vi "Open OPC UA Connection.vi"(8 "error in (no error)":errorcluster, 10 "OPC UA configuration":refnum<class "OPC UA configuration.lvclass">, 11 "OPC UA runtime in":refnum<class "OPC UA runtime.lvclass">) -> (0 "error out":errorcluster, 3 "OPC UA runtime out":refnum<class "OPC UA runtime.lvclass">)   [LabVIEW 2013, in "OPC UA runtime.lvclass"]
doc: "Opens connection to either an OPC UA Client or Server."
uses:
  OPC UA runtime.lvclass
  configuration/OPC UA configuration.lvclass
  configuration/OPC UA configuration.lvclass/OPC UA configuration.ctl
  OPC UA runtime.lvclass/OPC UA runtime.ctl
  configuration/Read Connection Configuration.vi
  configuration/Read Lines.vi
  <vilib>/NI/Tag Bus Module Framework/channel/TBM channel.lvclass
  <vilib>/opcua/NI OPC UA Server.lvlib
  <vilib>/opcua/NI OPC UA Client.lvlib
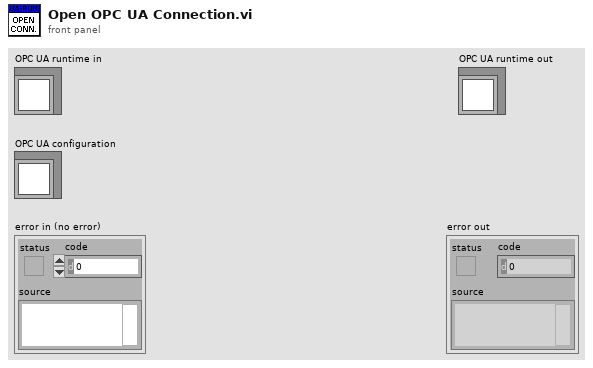
[diagram p1: front panel]
types:
  T1 = typedef "supported security policies.ctl" = cluster{"None":bool, "Sign with Basic128Rsa125":bool, "Sign and Encrypt with Basic128Rsa125":bool, "Sign with Basic256":bool, "Sign and Encrypt with Basic256":bool}
  T2 = cluster{"Client?":bool, "Server Certificates":cluster{"Relative Path?":bool, "Certificate Paths":path[], "Certificate Names":string[]}, "Client Certificates":cluster{"Relative Path?":bool, "Certificate Paths":path[], "Certificate Names":string[]}, "Client Configuration":cluster{"Server Endpoint URL":string, "Security Policy":cluster{"Message Mode":enum16{"None", "Sign", "Sign and Encrypt"}, "Security":enum16{"Basic256", "Basic128Rsa15"}}, "Username/Password":cluster{"Username":string, "Password":string}}, "Server Configuration":cluster{"Server Name":string, "TCP port (49580)":string, "Supported Security Policies":T1}}
  T3 = typedef "OPC UA configuration.lvclass/Line.ctl" = cluster{"channel":refnum<class "TBM channel.lvclass">, "Node Path":string, "OPC UA Data Type":T4}
  T4 = typedef "OPC UA configuration.lvclass/OPC UA Data Type.ctl" = u16
  T5 = cluster{"Relative Path?":bool, "Certificate Paths":path[], "Certificate Names":string[]}
  T6 = cluster{"Message Mode":enum16{"None", "Sign", "Sign and Encrypt"}, "Security":enum16{"Basic256", "Basic128Rsa15"}}
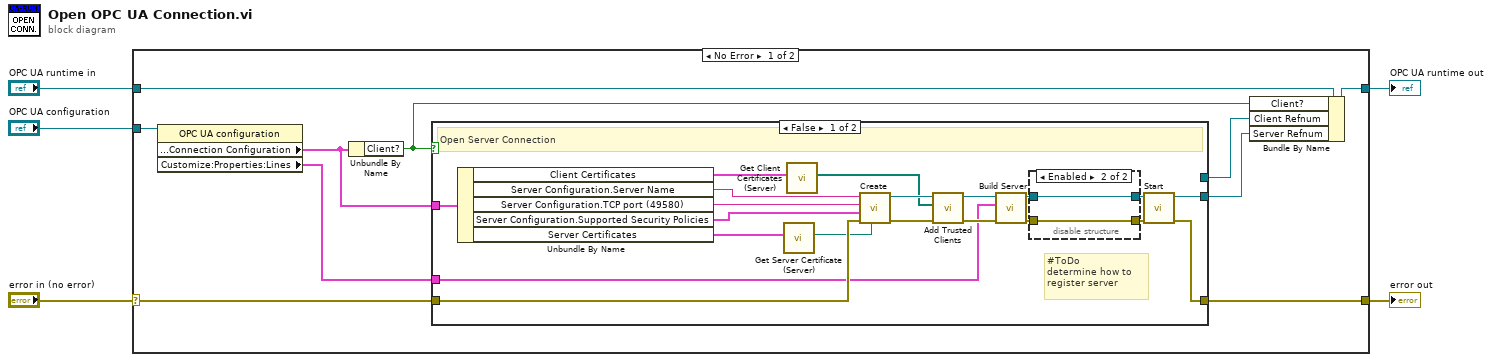
[diagram p0: block diagram]
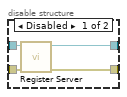
[diagram p2: hidden frame]
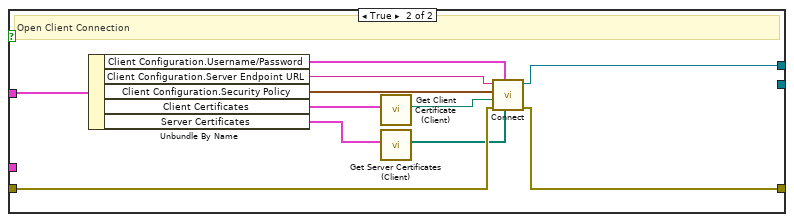
[diagram p3: hidden frame]
diagram:
  n1 = case shown="No Error" "error in (no error)" {
    selector: "error in (no error)" -> [w13 w54]
    tunnel: [w11 w54] -> w4
    tunnel: [w14 w53] -> w2
    tunnel: "OPC UA runtime in" -> [w15 w53]
    tunnel: "OPC UA configuration" -> [w8 _]
    frame No Error {
      n2 = property class="OPC UA configuration"(reference=w8) -> ("Customize:Properties:Connection Configuration"=w9:T2, "Customize:Properties:Lines"=w7:T3[])  [unwired: 1 in, 2 out]
      n3 = Unbundle By Name(w9) -> ("Client?"=w6:bool)
      n4 = case shown="False" w6 {
        tunnel: w9 -> [w35 w49]
        tunnel: w13 -> [w34 w52]
        tunnel: [w24 _] -> w12
        tunnel: [w25 w51] -> w11
        tunnel: [_ w50] -> w10
        tunnel: w7 -> [w17 _]
        frame False {
          # "#ToDo\ndetermine how to\nregister server"
          # "Open Server Connection"
          n5 = Unbundle By Name(w35) -> ("Client Certificates"=w27:T5, "Server Configuration.Server Name"=w31:string, "Server Configuration.TCP port (49580)"=w32:string, "Server Configuration.Supported Security Policies"=w33:T1, "Server Certificates"=w30:T5)
          n6 = call "Get Server Certificate (Server).vi"("Server Certificates"=w30) -> ("server certificate file"=w29:path)  [unwired: 10 in]
          n7 = call "Get Client Certificates (Server).vi"("Client Certificates"=w27) -> ("trusted client certificates"=w26:path[])  [unwired: 10 in]
          n8 = call <vilib>:"Create.vi"("server certificate file"=w29, "error in (no error)"=w34, "supported security policies (None)"=w33, "TCP port (49580)"=w32, "OPC UA server name"=w31) -> ("error out"=w16:errorcluster, "OPC UA server refnum out"=w28:refnum<k21>)  [unwired: 4 in, 1 out]
          n9 = call <vilib>:"Add Trusted Clients.vi"("error in (no error)"=w16, "trusted client certificates"=w26, "OPC UA server refnum in"=w28) -> ("error out"=w22:errorcluster, "OPC UA server refnum out"=w23:refnum<k21>)  [unwired: 7 in]
          n10 = call "Build Server.vi"("Error In"=w22, "Lines"=w17, "OPC UA server refnum in"=w23) -> ("Error Out"=w20:errorcluster, "OPC UA server refnum out"=w21:refnum<k21>)  [unwired: 7 in]
          n11 = disable-structure shown="Enabled" {
            disable-tunnel: w21 -> [w39 w41]
            disable-tunnel: w20 -> [w38 w40]
            disable-tunnel: [w37 w40] -> w19
            disable-tunnel: [w36 w41] -> w18
            frame Disabled {
              n12 = call <vilib>:"Register Server.vi"("error in (no error)"=w38, "OPC UA server refnum in"=w39) -> ("error out"=w37:errorcluster, "OPC UA server refnum out"=w36:refnum<k21>)  [unwired: 8 in]
            }
            frame Enabled {
            }
          }
          n13 = call <vilib>:"Start.vi"("error in (no error)"=w19, "OPC UA server refnum in"=w18) -> ("error out"=w25:errorcluster, "OPC UA server refnum out"=w24:refnum<k21>)  [unwired: 8 in]
        }
        frame True {
          # "Open Client Connection"
          n14 = Unbundle By Name(w49) -> ("Client Configuration.Username/Password"=w48:cluster{"Username":string, "Password":string}, "Client Configuration.Server Endpoint URL"=w47:string, "Client Configuration.Security Policy"=w46:T6, "Client Certificates"=w45:T5, "Server Certificates"=w43:T5)
          n15 = call "Get Client Certificate (Client).vi"("Client Certificates"=w45) -> ("client certificate file"=w44:path)  [unwired: 10 in]
          n16 = call "Get Server Certificates (Client).vi"("Server Certificates"=w43) -> ("trusted server certificates"=w42:path[])  [unwired: 10 in]
          n17 = call <vilib>:"Connect.vi"("trusted server certificates"=w42, "username/password"=w48, "error in (no error)"=w52, "client certificate file"=w44, "security policy"=w46, "server endpoint URL"=w47) -> ("error out"=w51:errorcluster, "OPC UA client refnum out"=w50:refnum<k21>)  [unwired: 3 in, 1 out]
        }
      }
      n18 = Bundle By Name(cluster=w15, "Client?"=w6, "Client Refnum"=w10, "Server Refnum"=w12) -> (w14:refnum<class "OPC UA runtime.lvclass">)
    }
    frame Error {
    }
  }
  "error out" <- w4
  "OPC UA runtime out" <- w2
